vi "Add Skipped.vi"(6 "Outcome Attributes":T1, 8 "Error In (No Error)":errorcluster, 9 "Text":string, 10 "Testcase Ref":refnum<k20>, 11 "File Ref In":refnum<k20>) -> (0 "Error Out":errorcluster, 2 "Testcase Ref Out":refnum<k20>, 3 "File Ref Out":refnum<k20>)   [LabVIEW 2013, in "JUnit API.lvlib"]
uses:
  JUnit API.lvlib
  Controls/Outcome Attributes.ctl
  <vilib>/NI/Simple XML/_polymorphics/Create Tag - Child with Text.vi
  <vilib>/xml/Close Reference(Node).vi
  <vilib>/NI/Simple XML/Simple XML.lvlib
  <vilib>/xml/NI_XML.lvlib
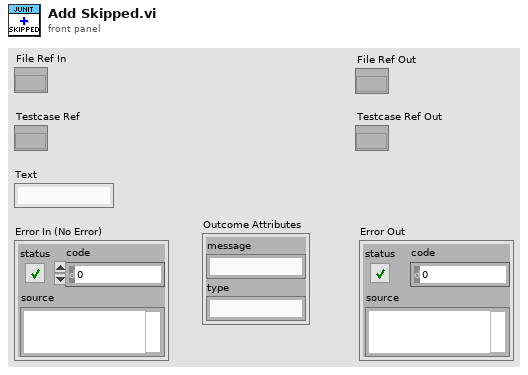
[diagram p1: front panel]
types:
  T1 = typedef "JUnit API.lvlib/Outcome Attributes.ctl" = cluster{"message":string, "type":string}
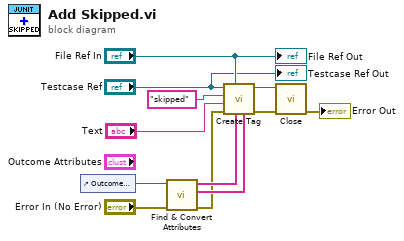
[diagram p0: block diagram]
diagram:
  n1 = control-ref of="Outcome Attributes"() -> (w1:refnum<vi>)
  n2 = call "Find & Convert Attributes.vi"("Error In"="Error In (No Error)", "Cluster in"=w1) -> ("Error Out"=w2:errorcluster, "Attribute Values"=w4:string[], "Attribute Names"=w5:string[])  [unwired: 7 in]
  n3 = call-poly <vilib>:"Create Tag.vi"("Attr Values"=w4, "Attr Names"=w5, "DOM document reference"="File Ref In", "error in (no error)"=w2, "Text Data"="Text", "Tag Name"="skipped", "Parent Element reference"="Testcase Ref") -> ("error out"=w7:errorcluster, "Child Element reference"=w8:refnum<k20>)  [unwired: 3 in]
  n4 = call-poly <vilib>:"Close.vi"("error in (no error)"=w7, "node"=w8) -> ("error out"=→"Error Out":errorcluster)  [unwired: 7 in]
  "File Ref Out" <- "File Ref In"
  "Testcase Ref Out" <- "Testcase Ref"
